vi "Process Incoming Messages by PDU F.vi"(0 "J1939 Cluster":T11, 1 "Scale Ref":T2, 2 "Data Ref":T1, 5 "CAN frame":T9 {"payload" format="%x"; "timestamp" format="%<%.7X\n%x>T"; "type" items=["CAN Data"=0, "CAN Remote"=1, "CAN Bus Error"=2, "CAN 2.0 Data"=8, "CAN FD Data"=16, "CAN FD+BRS Data"=24, "J1939 Data"=192, "Delay"=224, "Log Trigger"=225, "Start Trigger"=226]; "identifier" format="%x"}, 7 "ref in":T3, 9 "Addresses":u8[](array[numeric]), 11 "error in":errorcluster, 12 "Simulated Addresses LUT":variant) -> (15 "error out":errorcluster)   [LabVIEW 2015, in "J1939 Addon Engine.lvlib"]
uses:
  J1939 Addon Engine.lvlib
  Types/Setup Information Cluster.ctl
  <vilib>/xnet/xnet.llb/XNET Frame CAN.ctl
  <vilib>/xnet/xnet.llb/XNET Frame Type CAN.ctl
  Shared/J1939 Utilities/Types/CAN Outgoing Message Cluster.ctl
  Types/TP List References.ctl
  Types/BAM Buffer Connections List_Ref.ctl
  Types/TP Buffer Connection Cluster.ctl
  Types/Connection Mode Generation Connection Ref.ctl
  Types/Connection Mode Generation Connection Cluster.ctl
  Types/BAM Generation Connections List_Ref.ctl
  Types/BAM Generation Connection Cluster.ctl
  Types/Address Table Reference.ctl
  Types/RQST Lookup Table Reference.ctl
  Types/Conversion Lookup Table Reference.ctl
  Types/Data Lookup Table Reference.ctl
  Types/Datatable Lookup DVR.ctl
  Shared/J1939 Utilities/Types/PGN Fields Cluster.ctl
  Types/Simulated Settings.ctl
  Shared/Types/Compiled Simulated Settings.ctl
  Shared/Types/Monitor Settings.ctl
  <vilib>/NI Veristand/Custom Device API/Block Data Reference.ctl
  <vilib>/NI Veristand/Custom Device API/Data Reference.ctl
  Types/DTC FIFOs.ctl
  Types/TP Connections List State.ctl
  Types/Connection Mode Buffer Create New TP Connection State.ctl
  Types/Address Lookup Table Action.ctl
  Shared/Types/Address Lookup Table Data.ctl
  Shared/J1939 Utilities/SubVIs/Convert CAN Arb ID to J1939 ID.vi
  Shared/J1939 Utilities/SubVIs/Convert J1939 ID to CAN Arb ID.vi
  Shared/J1939 Utilities/SubVIs/Convert CAN Data (U32) to U8.vi
  Shared/J1939 Utilities/SubVIs/Acknowledgement.vi
  Buffer Connections List_Actions.vi
  TP Buffer Search for Connection (No PGN).vi
  TP Buffer Add New Data Packet to Connection.vi
  TP Buffer Convert Connection Info to CAN Frame.vi
  TP Buffer Create New TP Connection.vi
  Shared/J1939 Utilities/SubVIs/TP.CM EndofMsgACK.vi
  Shared/J1939 Utilities/SubVIs/TP.CM CTS.vi
  Shared/J1939 Utilities/SubVIs/TP.Conn Abort.vi
  Connection Mode Generation Connections List_Actions.vi
  Connection Mode Generation Search for Connection (Remote Message).vi
  TP Buffer Search for Connection.vi
  Connection Mode Generation CTS Received.vi
  Convert Data to DTC Frame.vi
  Conversion Lookup Table Get Conversion Parameter.vi
  Data Lookup Table Get Signals (Range).vi
  Shared/J1939 Utilities/SubVIs/Convert PGN + SA to J1939 ID.vi
  Address Lookup Table.vi
  BAM Buffer Connections List.vi
  Connection Mode Generation Connections List.vi
  <vilib>/xnet/xnet.llb/XNET Convert.vi
  <vilib>/xnet/xnet.llb/XNET Convert (Signal to Frame Raw).vi
  Data Lookup Table.vi
  Conversion Lookup Table.vi
  RQST Lookup Table.vi
  Shared/J1939 Utilities/J1939 Utilities.lvlib
  Shared/J1939 Addon Shared.lvlib
  <vilib>/NI VeriStand/Custom Device API/Custom Device API.lvlib
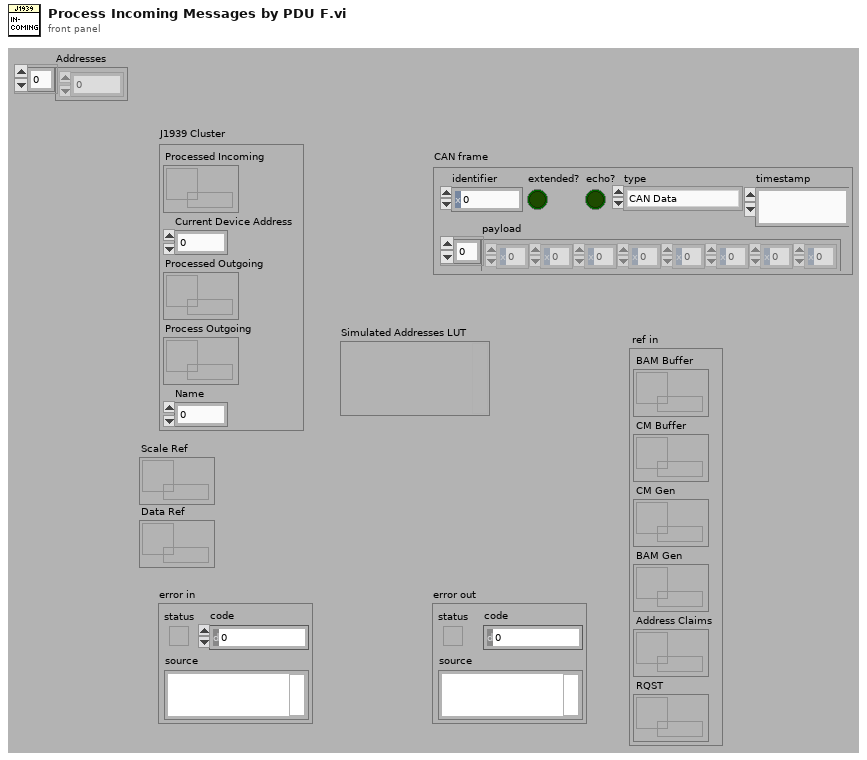
[diagram p1: front panel]
types:
  T1 = typedef "J1939 Addon Engine.lvlib/Data Lookup Table Reference.ctl" = refnum<data-value>
  T2 = typedef "J1939 Addon Engine.lvlib/Conversion Lookup Table Reference.ctl" = refnum<data-value>
  T3 = typedef "J1939 Addon Engine.lvlib/TP List References.ctl" = cluster{"BAM Buffer":T4, "CM Buffer":T4, "CM Gen":T5, "BAM Gen":T6, "Address Claims":T7, "RQST":T8}
  T4 = typedef "J1939 Addon Engine.lvlib/BAM Buffer Connections List_Ref.ctl" = refnum<data-value>
  T5 = typedef "J1939 Addon Engine.lvlib/Connection Mode Generation Connection Ref.ctl" = refnum<data-value>
  T6 = typedef "J1939 Addon Engine.lvlib/BAM Generation Connections List_Ref.ctl" = refnum<data-value>
  T7 = typedef "J1939 Addon Engine.lvlib/Address Table Reference.ctl" = refnum<data-value>
  T8 = typedef "J1939 Addon Engine.lvlib/RQST Lookup Table Reference.ctl" = refnum<data-value>
  T9 = typedef "XNET Frame CAN.ctl" = cluster{"timestamp":timestamp, "payload":u8[], "identifier":u32, "type":T10, "extended?":bool, "echo?":bool}
  T10 = typedef "XNET Frame Type CAN.ctl" = u8
  T11 = typedef "J1939 Addon Engine.lvlib/Setup Information Cluster.ctl" = cluster{"Processed Incoming":refnum<queue>, "Current Device Address":u8, "Processed Outgoing":refnum<queue>, "Process Outgoing":refnum<queue>, "Name":u64}
  T12 = typedef "J1939 Addon Shared.lvlib/J1939 Utilities.lvlib/Message Types.ctl" = enum8{"PDU 1", "RQST2", "XFER", "ACKM", "RQST", "TP.DT - RTS/CTS", "TP.DT - BAM", "TP.CM - RTS", "TP.CM - CTS", "TP.CM - EndofMsgACK", "TP.CM - BAM", "TP.CM - Abort", "TP.CM - Error", "ACL", "Proprietary A", "PDU 2", "Proprietary B", "Error"}
  T13 = typedef "J1939 Addon Engine.lvlib/Simulated Settings.ctl" = cluster{"Simulated Addresses":T14, "FIFOs":T18}
  T14 = typedef "J1939 Addon Shared.lvlib/Compiled Simulated Settings.ctl" = cluster{"J1939 XNET Settings":T15, "DM1 Data":T16[], "DM1 Data":dbl[], "DM1 Enable?":T16[], "DM1 Enable?":dbl[], "DM2 Data":T16[], "DM2 Data":dbl[], "DM2 Enable?":T16[], "DM2 Enable?":dbl[]}
  T15 = typedef "J1939 Addon Shared.lvlib/Monitor Settings.ctl" = cluster{"J1939 Network Address":u8, "Name":u64}
  T16 = typedef "Custom Device API.lvlib/Block Data Reference.ctl" = cluster{"Data Reference":T17, "Offset":u64, "Length":u64}
  T17 = typedef "Custom Device API.lvlib/Data Reference.ctl" = i32
  T18 = typedef "J1939 Addon Engine.lvlib/DTC FIFOs.ctl" = cluster{"DM1 Data":refnum<k33>, "DM1 Enable?":refnum<k33>, "DM2 Data":refnum<k33>, "DM2 Enable?":refnum<k33>, "DM1 Reset?":refnum<k33>, "DM2 Reset?":refnum<k33>}
  T19 = typedef "J1939 Addon Shared.lvlib/J1939 Utilities.lvlib/PGN Fields Cluster.ctl" = cluster{"Reserved Bit":u8, "Data page":u8, "PDU Format":u8, "PDU Specific":u8}
  T20 = typedef "J1939 Addon Shared.lvlib/J1939 Utilities.lvlib/CAN Outgoing Message Cluster.ctl" = cluster{"Identifier":u32, "Data":u8[]}
  T21 = typedef "J1939 Addon Engine.lvlib/TP Connections List State.ctl" = enum16{"Add", "Update", "Get", "Remove", "Initialize"}
  T22 = typedef "J1939 Addon Engine.lvlib/Connection Mode Buffer Create New TP Connection State.ctl" = enum8{"Find Connection", "Create Connection", "Create CTS Frame", "Abort New Connection"}
  T23 = typedef "J1939 Addon Shared.lvlib/Address Lookup Table Data.ctl" = cluster{"Name":u8[], "Address":u8}
  T24 = typedef "J1939 Addon Engine.lvlib/Address Lookup Table Action.ctl" = enum16{"Initialize", "Add", "Get", "Remove", "Get All"}
  T25 = typedef "J1939 Addon Engine.lvlib/RQST Lookup Table Cluster.ctl" = cluster{"Response Q":refnum<queue>, "Request PGN":u32}
  T26 = typedef "J1939 Addon Shared.lvlib/J1939 Utilities.lvlib/Convert CAN Data (U8) Cluster.ctl" = cluster{"Byte 1":u8, "Byte 2":u8, "Byte 3":u8, "Byte 4":u8, "Byte 5":u8, "Byte 6":u8, "Byte 7":u8, "Byte 8":u8}
  T27 = typedef "J1939 Addon Engine.lvlib/TP Buffer Connection Cluster.ctl" = cluster{"Source Address":u8, "Destination Address":u8, "PGN":u32, "Arb ID":u32, "CAN Conversion Index":u32, "Total Expected Bytes":u16, "Total Expected Packets":u8, "Number of Packets Read":u8, "Start Time":u32, "Packets (U8)":u8[], "Timestamp":timestamp}
  T28 = typedef "J1939 Addon Engine.lvlib/Connection Mode Generation Connection Cluster.ctl" = cluster{"Total Packets":u8, "Current Packet to Generate":u8, "Packets":T20[], "Previous Time Stamp":u32, "Total Bytes":u16, "Packet Identifier [PDU S + SA]":u16, "Number of Packets to Generate":u8, "PGN":u32}
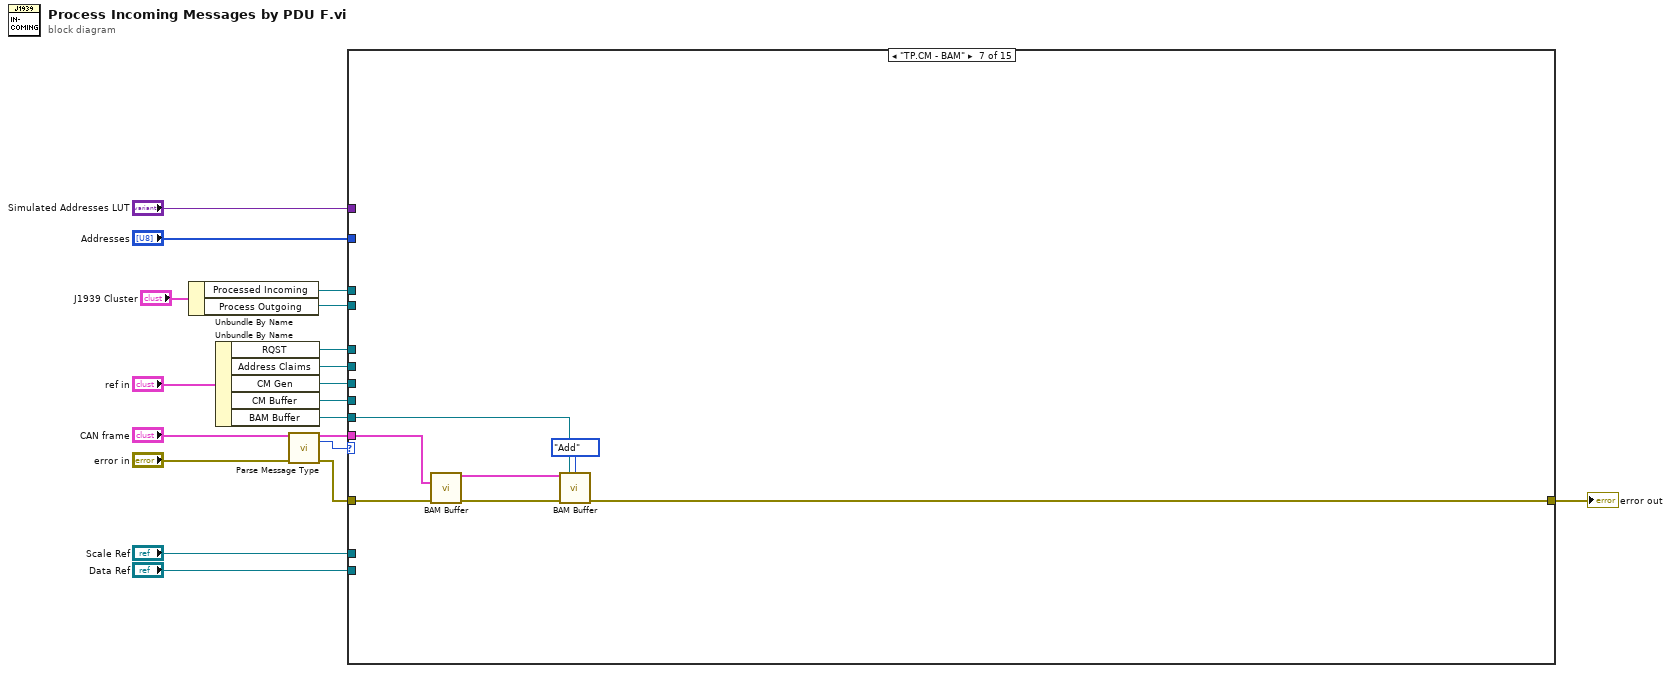
[diagram p0: block diagram]
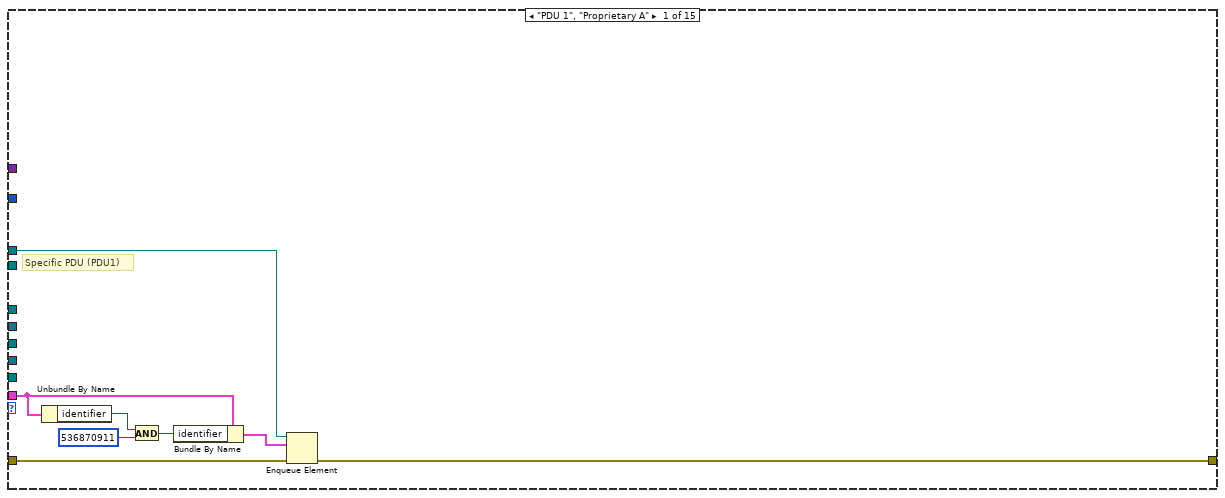
[diagram p2: hidden frame]
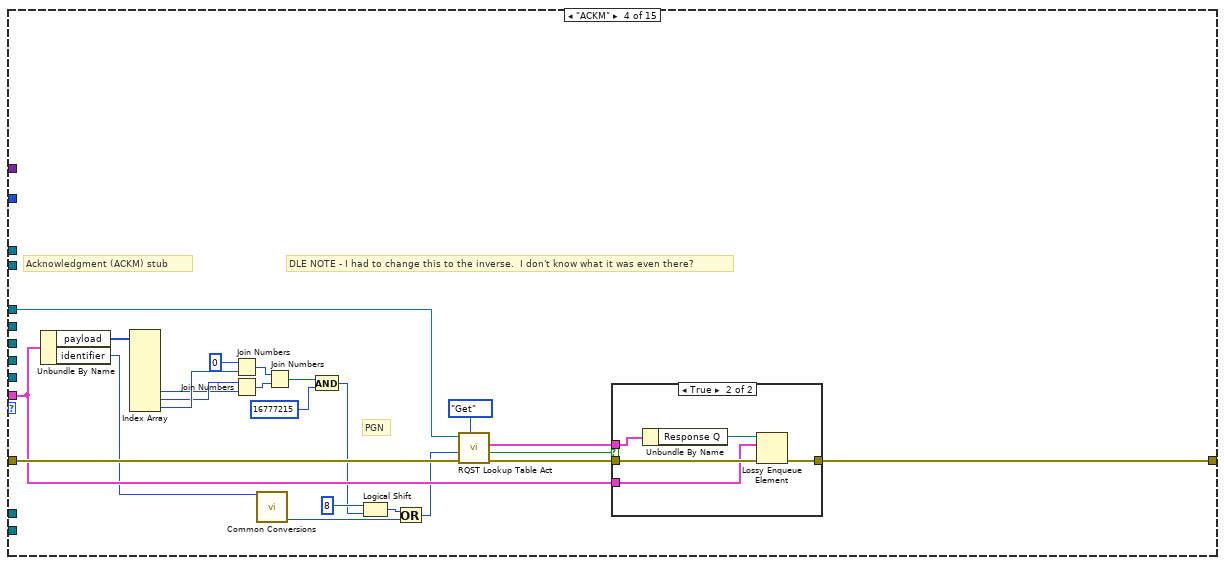
[diagram p5: hidden frame]
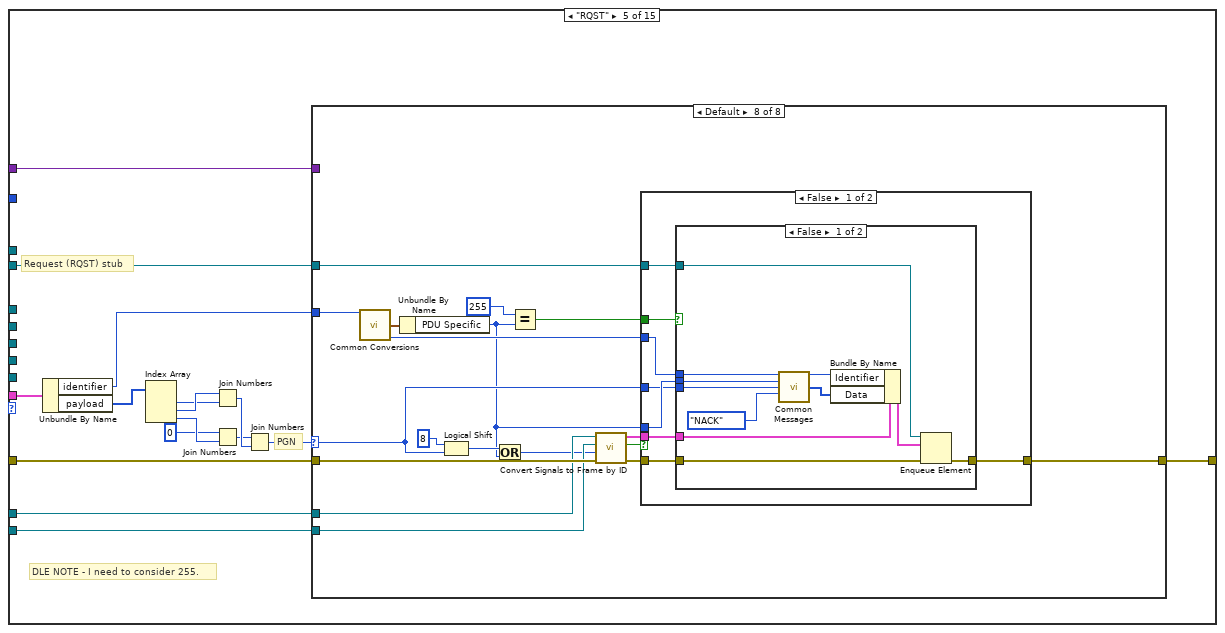
[diagram p7: hidden frame]
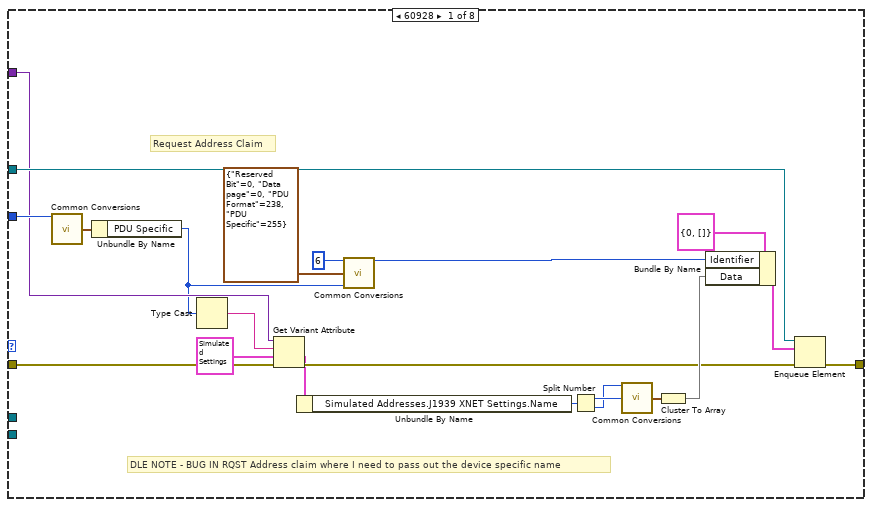
[diagram p8: hidden frame]
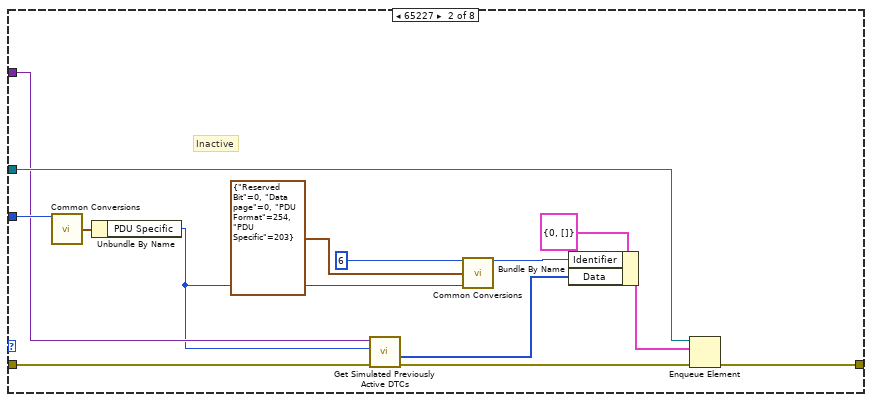
[diagram p9: hidden frame]
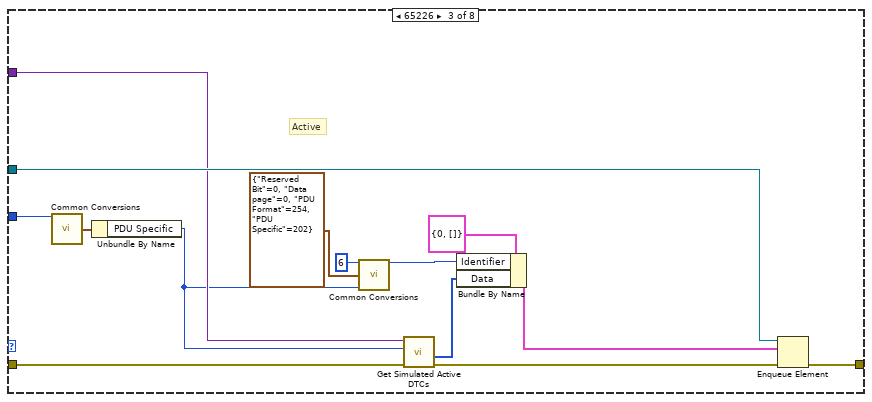
[diagram p10: hidden frame]
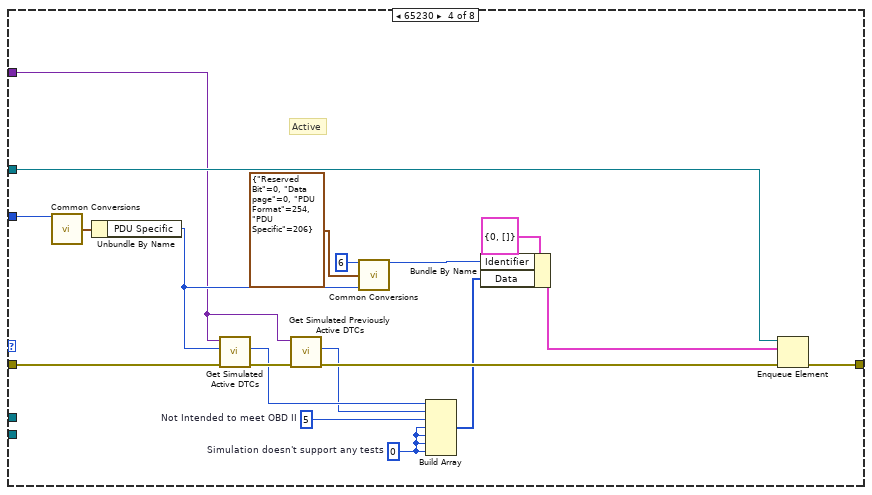
[diagram p11: hidden frame]
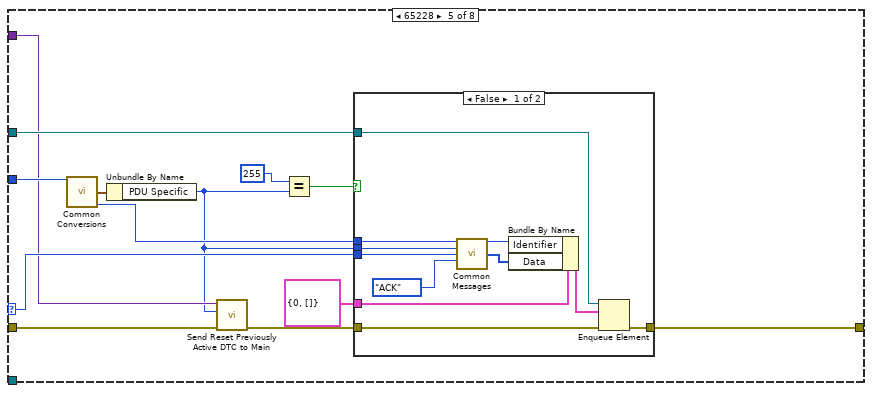
[diagram p12: hidden frame]
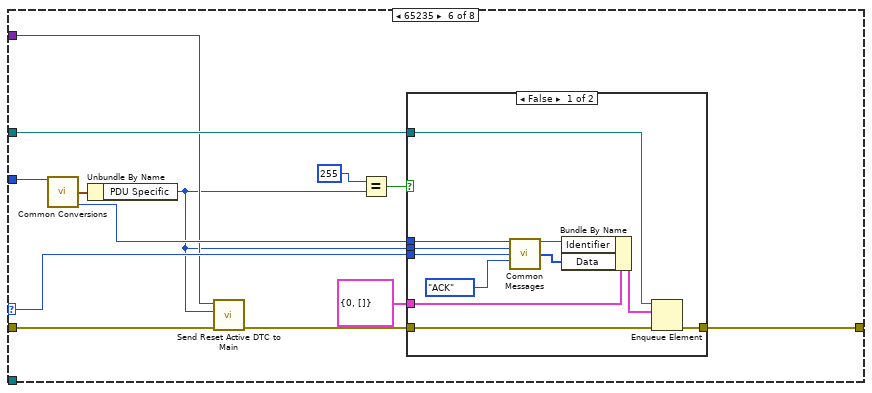
[diagram p14: hidden frame]
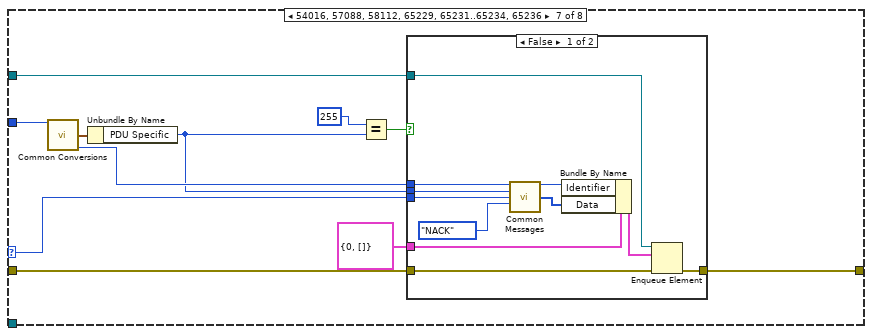
[diagram p16: hidden frame]
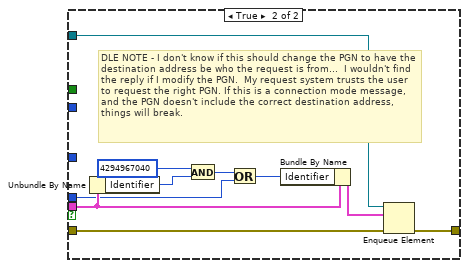
[diagram p19: hidden frame]
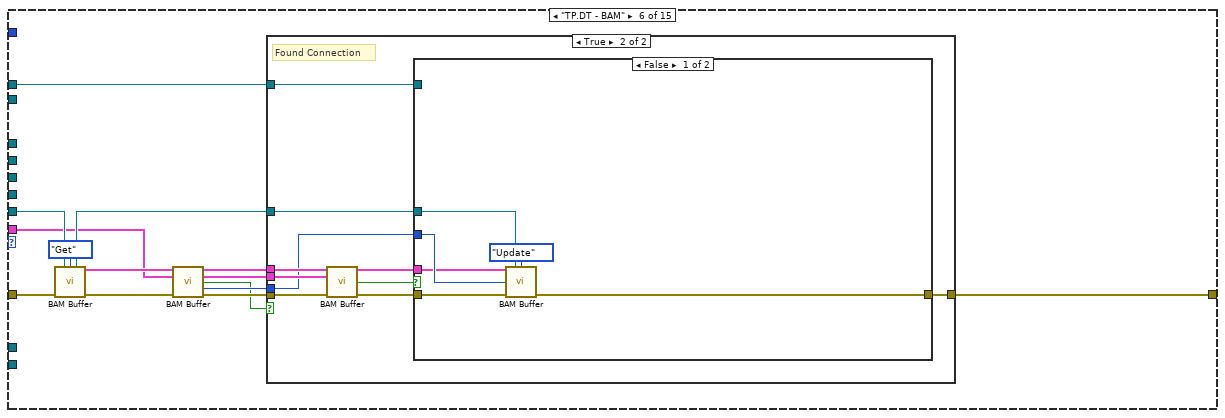
[diagram p20: hidden frame]
diagram:
  n1 = Unbundle By Name("J1939 Cluster") -> ("Processed Incoming"=w13:refnum<queue>, "Process Outgoing"=w12:refnum<queue>)
  n2 = Unbundle By Name("ref in") -> ("RQST"=w6:T8, "Address Claims"=w7:T7, "CM Gen"=w8:T5, "CM Buffer"=w9:T4, "BAM Buffer"=w10:T4)
  n3 = call "Parse Message Type.vi"("CAN frame"="CAN frame", "error in"="error in") -> ("CAN frame"=w16:T9, "State"=w15:T12, "error out"=w17:errorcluster)  [unwired: 1 in, 10 out]
  n4 = case shown="\"TP.CM - BAM\"" w15 {
    tunnel: w17 -> [w27 w28 w29 w39 w65 w270 w311 w327 w394 w496 w537 w553 w589 w601 w607]
    tunnel: [w26 w28 w29 w40 w66 w272 w308 w320 w393 w495 w536 w554 w582 w602 w607] -> w19
    tunnel: w16 -> [w22 _ _ w38 w74 w264 w305 w314 w390 w484 w527 w544 w580 w599 _]
    tunnel: w13 -> [w25 _ _ _ _ w267 _ w318 _ _ _ _ w579 w600 _]
    tunnel: w12 -> [_ _ _ _ w64 _ _ w317 w392 _ _ _ _ _ _]
    tunnel: w10 -> [_ _ _ _ _ w266 w306 _ _ _ _ _ _ _ _]
    tunnel: w9 -> [_ _ _ _ _ _ _ w316 w391 w483 _ w547 _ _ _]
    tunnel: w8 -> [_ _ _ _ _ _ _ _ _ w486 w529 w545 _ _ _]
    tunnel: w7 -> [_ _ _ _ _ _ _ _ _ _ _ _ w587 _ _]
    tunnel: w6 -> [_ _ _ w30 _ _ _ _ _ _ _ _ _ _ _]
    tunnel: "Scale Ref" -> [_ _ _ _ w62 _ _ _ _ _ _ _ _ _ _]
    tunnel: "Data Ref" -> [_ _ _ _ w61 _ _ _ _ _ _ _ _ _ _]
    tunnel: "Addresses" -> [_ _ _ _ _ _ _ w312 w389 _ _ _ _ _ _]
    tunnel: "Simulated Addresses LUT" -> [_ _ _ _ w59 _ _ _ _ _ _ _ _ _ _]
    frame "PDU 1", "Proprietary A" {
      # "Specific PDU (PDU1)"
      n5 = Unbundle By Name(w22) -> ("identifier"=w24:u32)
      n6 = And(x=w24, y=u32 536870911) -> (x .and. y?=w20:u32)
      n7 = Bundle By Name(cluster=w22, "identifier"=w20) -> (w21:T9)
      n8 = Enqueue Element(queue=w25, element=w21, error in (no error)=w27) -> (error out=w26:errorcluster)  [unwired: 3 out]
    }
    frame "RQST2" {
      # "Request2 (RQST2) Stub"
    }
    frame "XFER" {
      # "Transfer (XFER) Stub"
    }
    frame "ACKM" {
      # "DLE NOTE - I had to change this to the inverse.  I don't know what it was even there?"
      # "PGN"
      # "Acknowledgment (ACKM) stub"
      n9 = Unbundle By Name(w38) -> ("payload"=w52:u8[], "identifier"=w35:u32)
      n10 = Index Array(array=w52) -> (element #6=w49:u8, element #7=w50:u8, element #8=w51:u8)  [unwired: 8 in, 5 out]
      n11 = Join Numbers(hi=u8 0, lo=w51) -> ((hi.lo)=w48:u16)
      n12 = Join Numbers(hi=w50, lo=w49) -> ((hi.lo)=w47:u16)
      n13 = call-poly "Common Conversions.vi"("Arb ID"=w35) -> ("Source Address"=w34:u8)  [unwired: 11 in, 3 out]
      n14 = Join Numbers(hi=w48, lo=w47) -> ((hi.lo)=w46:u32)
      n15 = And(x=w46, y=u32 16777215 ("x")) -> (x .and. y?=w33:u32)
      n16 = Logical Shift(y=i8 8, x=w33) -> (x << y=w37:u32)
      n17 = Or(x=w37, y=w34) -> (x .or. y?=w32:u32)
      n18 = call "RQST Lookup Table Act.vi"("Action"=enum16{"Initialize", "Add", "Get", "Remove"}."Get", "error in (no error)"=w39, "ID"=w32, "Rqst LUT"=w30) -> ("error out"=w31:errorcluster, "Found?"=w42:bool, "Data"=w41:T25)  [unwired: 4 in, 1 out]
      n19 = case shown="True" w42 {
        tunnel: w41 -> [_ w57]
        tunnel: w31 -> [w53 w58]
        tunnel: w38 -> [_ w55]
        tunnel: [w53 w54] -> w40
        frame False {
        }
        frame True {
          n20 = Unbundle By Name(w57) -> ("Response Q"=w56:refnum<queue>)
          n21 = Lossy Enqueue Element(queue=w56, element=w55, error in (no error)=w58) -> (error out=w54:errorcluster)  [unwired: 3 out]
        }
      }
    }
    frame "RQST" {
      # "DLE NOTE - I need to consider 255."
      # "PGN"
      # "Request (RQST) stub"
      n22 = Unbundle By Name(w74) -> ("identifier"=w63:u32, "payload"=w73:u8[])
      n23 = Index Array(array=w73) -> (element #1=w60:u8, element #2=w72:u8, element #3=w71:u8)  [unwired: 3 in]
      n24 = Join Numbers(hi=w72, lo=w60) -> ((hi.lo)=w69:u16)
      n25 = Join Numbers(hi=u8 0, lo=w71) -> ((hi.lo)=w68:u16)
      n26 = Join Numbers(hi=w68, lo=w69) -> ((hi.lo)=w67:u32)
      n27 = case shown="Default" w67 {
        selector: w67 -> [_ _ _ _ w149 w174 w197 w223]
        tunnel: [w91 w102 w117 w136 w150 w172 w195 w224] -> w66
        tunnel: w65 -> [w78 w98 w111 w132 w146 w171 w193 w233]
        tunnel: w64 -> [w89 w101 w116 w135 w151 w175 w198 w225]
        tunnel: w63 -> [w83 w108 w122 w141 w154 w173 w196 w226]
        tunnel: w62 -> [_ _ _ _ _ _ _ w232]
        tunnel: w61 -> [_ _ _ _ _ _ _ w231]
        tunnel: w59 -> [w80 w100 w113 w129 w144 w169 _ _]
        frame 60928 {
          # "DLE NOTE - BUG IN RQST Address claim where I need to pass out the device specific name"
          # "Request Address Claim"
          n28 = call-poly "Common Conversions.vi"("Arb ID"=w83) -> ("PGN Fields"=w84:T19)  [unwired: 11 in, 3 out]
          n29 = Unbundle By Name(w84) -> ("PDU Specific"=w79:u8)
          n30 = Type Cast(x=w79) -> (*(type *) &x=w81:string)  [unwired: 1 in]
          n31 = Get Variant Attribute(Variant=w80, name=w81, default value (empty Variant)=T13 {"Simulated Addresses"={"J1939 XNET Settings"={"J1939 Network Address"=0, "Name"=0}, "DM1 Data"=[], "DM1 Data"=[], "DM1 Enable?"=[], "DM1 Enable?"=[], "DM2 Data"=[], "DM2 Data"=[], "DM2 Enable?"=[], "DM2 Enable?"=[]}, "FIFOs"={"DM1 Data"=refnum, "DM1 Enable?"=refnum, "DM2 Data"=refnum, "DM2 Enable?"=refnum, "DM1 Reset?"=refnum, "DM2 Reset?"=refnum}} ("Cluster"), error in=w78) -> (value=w76:T13, error out=w77:errorcluster)  [unwired: 2 out]
          n32 = Unbundle By Name(w76) -> ("Simulated Addresses.J1939 XNET Settings.Name"=w75:u64)
          n33 = call-poly "Common Conversions.vi"("Priority"=u8 6, "PGN Fields"=T19 {"Reserved Bit"=0, "Data page"=0, "PDU Format"=238, "PDU Specific"=255}, "Source Address"=w79) -> ("ID"=w93:u32)  [unwired: 2 in, 10 out]
          n34 = Split Number(x=w75) -> (hi(x)=w87:u32, lo(x)=w86:u32)
          n35 = call-poly "Common Conversions.vi"("Data 0-3"=w86, "Data 4-7"=w87) -> ("Byte Cluster"=w88:T26)  [unwired: 13 in]
          n36 = Cluster To Array(cluster=w88) -> (array=w85:u8[])
          n37 = Bundle By Name(cluster=T20 {"Identifier"=0, "Data"=[]} ("Data to Send"), "Identifier"=w93, "Data"=w85) -> (w90:T20)
          n38 = Enqueue Element(queue=w89, element=w90, error in (no error)=w77) -> (error out=w91:errorcluster)  [unwired: 1 in, 2 out]
        }
        frame 65227 {
          # "Inactive"
          n39 = call-poly "Common Conversions.vi"("Arb ID"=w108) -> ("PGN Fields"=w109:T19)  [unwired: 11 in, 3 out]
          n40 = Unbundle By Name(w109) -> ("PDU Specific"=w99:u8)
          n41 = call "Get Simulated Previously Active DTCs.vi"("error in (no error)"=w98, "Address"=w99, "Simulated Addresses LUT"=w100) -> ("error out"=w97:errorcluster, "DTC Frame"=w96:u8[])  [unwired: 5 in, 2 out]
          n42 = call-poly "Common Conversions.vi"("Priority"=u8 6, "PGN Fields"=T19 {"Reserved Bit"=0, "Data page"=0, "PDU Format"=254, "PDU Specific"=203}, "Source Address"=w99) -> ("ID"=w105:u32)  [unwired: 2 in, 10 out]
          n43 = Bundle By Name(cluster=T20 {"Identifier"=0, "Data"=[]} ("Data to Send"), "Identifier"=w105, "Data"=w96) -> (w107:T20)
          n44 = Enqueue Element(queue=w101, element=w107, error in (no error)=w97) -> (error out=w102:errorcluster)  [unwired: 1 in, 2 out]
        }
        frame 65226 {
          # "Active"
          n45 = call-poly "Common Conversions.vi"("Arb ID"=w122) -> ("PGN Fields"=w123:T19)  [unwired: 11 in, 3 out]
          n46 = Unbundle By Name(w123) -> ("PDU Specific"=w112:u8)
          n47 = call-poly "Common Conversions.vi"("Priority"=u8 6, "PGN Fields"=T19 {"Reserved Bit"=0, "Data page"=0, "PDU Format"=254, "PDU Specific"=202}, "Source Address"=w112) -> ("ID"=w119:u32)  [unwired: 2 in, 10 out]
          n48 = call "Get Simulated Active DTCs.vi"("error in (no error)"=w111, "Address"=w112, "Simulated Addresses LUT"=w113) -> ("error out"=w114:errorcluster, "DTC Frame"=w110:u8[])  [unwired: 5 in, 2 out]
          n49 = Bundle By Name(cluster=T20 {"Identifier"=0, "Data"=[]} ("Data to Send"), "Identifier"=w119, "Data"=w110) -> (w121:T20)
          n50 = Enqueue Element(queue=w116, element=w121, error in (no error)=w114) -> (error out=w117:errorcluster)  [unwired: 1 in, 2 out]
        }
        frame 65230 {
          w125 = u8 0  # Simulation doesn't support any tests
          w126 = u8 5  # Not Intended to meet OBD II
          # "Active"
          n51 = call-poly "Common Conversions.vi"("Arb ID"=w141) -> ("PGN Fields"=w142:T19)  [unwired: 11 in, 3 out]
          n52 = Unbundle By Name(w142) -> ("PDU Specific"=w133:u8)
          n53 = call "Get Simulated Active DTCs.vi"("error in (no error)"=w132, "Address"=w133, "Simulated Addresses LUT"=w129) -> ("error out"=w131:errorcluster, "# of Enabled"=w128:u8)  [unwired: 5 in, 2 out]
          n54 = call "Get Simulated Previously Active DTCs.vi"("error in (no error)"=w131, "Simulated Addresses LUT"=w129) -> ("error out"=w130:errorcluster, "# of Enabled"=w127:u8)  [unwired: 6 in, 2 out]
          n55 = call-poly "Common Conversions.vi"("Priority"=u8 6, "PGN Fields"=T19 {"Reserved Bit"=0, "Data page"=0, "PDU Format"=254, "PDU Specific"=206}, "Source Address"=w133) -> ("ID"=w138:u32)  [unwired: 2 in, 10 out]
          n56 = Build Array(w128, w127, w126, w125, w125, w125, w125) -> (w124:u8[])
          n57 = Bundle By Name(cluster=T20 {"Identifier"=0, "Data"=[]} ("Data to Send"), "Identifier"=w138, "Data"=w124) -> (w140:T20)
          n58 = Enqueue Element(queue=w135, element=w140, error in (no error)=w130) -> (error out=w136:errorcluster)  [unwired: 1 in, 2 out]
        }
        frame 65228 {
          n59 = call-poly "Common Conversions.vi"("Arb ID"=w154) -> ("PGN Fields"=w155:T19, "Source Address"=w148:u8)  [unwired: 11 in, 2 out]
          n60 = Unbundle By Name(w155) -> ("PDU Specific"=w143:u8)
          n61 = call "Send Reset Previously Active DTC to Main.vi"("error in (no error)"=w146, "Address"=w143, "Simulated Addresses LUT"=w144) -> ("error out"=w145:errorcluster)  [unwired: 7 in, 1 out]
          n62 = Equal?(x=u8 255 ("y"), y=w143) -> (x = y?=w152:bool)
          n63 = case shown="False" w152 {
            tunnel: w145 -> [w166 w167]
            tunnel: [w165 w167] -> w150
            tunnel: w151 -> [w164 _]
            tunnel: w148 -> [w163 _]
            tunnel: w143 -> [w162 _]
            tunnel: w149 -> [w161 _]
            tunnel: T20 {"Identifier"=0, "Data"=[]} ("Frame") -> [w159 _]
            frame False {
              n64 = call-poly "Common Messages.vi"("Destination Address"=w163, "Source Address"=w162, "PGN"=w161, "Control Byte"=enum8{"ACK", "NACK", "Access Denied"}."ACK") -> ("Arb ID"=w158:u32, "Data"=w157:u8[])  [unwired: 10 in]
              n65 = Bundle By Name(cluster=w159, "Identifier"=w158, "Data"=w157) -> (w156:T20)
              n66 = Enqueue Element(queue=w164, element=w156, error in (no error)=w166) -> (error out=w165:errorcluster)  [unwired: 3 out]
            }
            frame True {
            }
          }
        }
        frame 65235 {
          n67 = call-poly "Common Conversions.vi"("Arb ID"=w173) -> ("PGN Fields"=w180:T19, "Source Address"=w177:u8)  [unwired: 11 in, 2 out]
          n68 = Unbundle By Name(w180) -> ("PDU Specific"=w168:u8)
          n69 = call "Send Reset Active DTC to Main.vi"("error in (no error)"=w171, "Address"=w168, "Simulated Addresses LUT"=w169) -> ("error out"=w170:errorcluster)  [unwired: 7 in, 1 out]
          n70 = Equal?(x=u8 255 ("y"), y=w168) -> (x = y?=w178:bool)
          n71 = case shown="False" w178 {
            tunnel: w170 -> [w191 w192]
            tunnel: [w190 w192] -> w172
            tunnel: w175 -> [w189 _]
            tunnel: w177 -> [w188 _]
            tunnel: w168 -> [w187 _]
            tunnel: w174 -> [w186 _]
            tunnel: T20 {"Identifier"=0, "Data"=[]} ("Frame") -> [w184 _]
            frame False {
              n72 = call-poly "Common Messages.vi"("Destination Address"=w188, "Source Address"=w187, "PGN"=w186, "Control Byte"=enum8{"ACK", "NACK", "Access Denied"}."ACK") -> ("Arb ID"=w183:u32, "Data"=w182:u8[])  [unwired: 10 in]
              n73 = Bundle By Name(cluster=w184, "Identifier"=w183, "Data"=w182) -> (w181:T20)
              n74 = Enqueue Element(queue=w189, element=w181, error in (no error)=w191) -> (error out=w190:errorcluster)  [unwired: 3 out]
            }
            frame True {
            }
          }
        }
        frame 54016, 57088, 58112, 65229, 65231..65234, 65236 {
          n75 = call-poly "Common Conversions.vi"("Arb ID"=w196) -> ("PGN Fields"=w203:T19, "Source Address"=w200:u8)  [unwired: 11 in, 2 out]
          n76 = Unbundle By Name(w203) -> ("PDU Specific"=w194:u8)
          n77 = Equal?(x=u8 255 ("y"), y=w194) -> (x = y?=w201:bool)
          n78 = case shown="False" w201 {
            tunnel: w193 -> [w214 w215]
            tunnel: [w213 w215] -> w195
            tunnel: w198 -> [w212 _]
            tunnel: w200 -> [w211 _]
            tunnel: w194 -> [w210 _]
            tunnel: w197 -> [w209 _]
            tunnel: T20 {"Identifier"=0, "Data"=[]} ("Frame") -> [w207 _]
            frame False {
              n79 = call-poly "Common Messages.vi"("Destination Address"=w211, "Source Address"=w210, "PGN"=w209, "Control Byte"=enum8{"ACK", "NACK", "Access Denied"}."NACK") -> ("Arb ID"=w206:u32, "Data"=w205:u8[])  [unwired: 10 in]
              n80 = Bundle By Name(cluster=w207, "Identifier"=w206, "Data"=w205) -> (w204:T20)
              n81 = Enqueue Element(queue=w212, element=w204, error in (no error)=w214) -> (error out=w213:errorcluster)  [unwired: 3 out]
            }
            frame True {
            }
          }
        }
        frame Default {
          n82 = call-poly "Common Conversions.vi"("Arb ID"=w226) -> ("PGN Fields"=w222:T19, "Source Address"=w219:u8)  [unwired: 11 in, 2 out]
          n83 = Unbundle By Name(w222) -> ("PDU Specific"=w216:u8)
          n84 = Logical Shift(y=i8 8, x=w223) -> (x << y=w218:u32)
          n85 = Or(x=w218, y=w216) -> (x .or. y?=w217:u32)
          n86 = Equal?(x=u8 255 ("y"), y=w216) -> (x = y?=w220:bool)
          n87 = call "Convert Signals to Frame by ID.vi"("error in (no error)"=w233, "ID"=w217, "Data Ref"=w231, "Scale Ref"=w232) -> ("error out"=w227:errorcluster, "Found?"=w228:bool, "Frame"=w229:T20)  [unwired: 5 in]
          n88 = case shown="False" w228 {
            tunnel: w229 -> [w235 w263]
            tunnel: w216 -> [w237 w261]
            tunnel: [w240 w256] -> w224
            tunnel: w227 -> [w241 w257]
            tunnel: w219 -> [w238 _]
            tunnel: w225 -> [w239 w258]
            tunnel: w223 -> [w236 _]
            tunnel: w220 -> [w234 _]
            frame False {
              n89 = case shown="False" w234 {
                tunnel: w241 -> [w252 w253]
                tunnel: [w251 w253] -> w240
                tunnel: w239 -> [w250 _]
                tunnel: w238 -> [w249 _]
                tunnel: w237 -> [w248 _]
                tunnel: w236 -> [w247 _]
                tunnel: w235 -> [w245 _]
                frame False {
                  n90 = call-poly "Common Messages.vi"("Destination Address"=w249, "Source Address"=w248, "PGN"=w247, "Control Byte"=enum8{"ACK", "NACK", "Access Denied"}."NACK") -> ("Arb ID"=w244:u32, "Data"=w243:u8[])  [unwired: 10 in]
                  n91 = Bundle By Name(cluster=w245, "Identifier"=w244, "Data"=w243) -> (w242:T20)
                  n92 = Enqueue Element(queue=w250, element=w242, error in (no error)=w252) -> (error out=w251:errorcluster)  [unwired: 3 out]
                }
                frame True {
                }
              }
            }
            frame True {
              # "DLE NOTE - I don't know if this should change the PGN to have the destination address be who the request is from...  I wouldn't find the reply if I modify the PGN.  My request system trusts the user to request the right PGN. If this is a connection mode message, and the PGN doesn't include the correct destination address, things will break."
              n93 = Unbundle By Name(w263) -> ("Identifier"=w262:u32)
              n94 = And(x=u32 4294967040 ("y"), y=w262) -> (x .and. y?=w254:u32)
              n95 = Or(x=w254, y=w261) -> (x .or. y?=w260:u32)
              n96 = Bundle By Name(cluster=w263, "Identifier"=w260) -> (w259:T20)
              n97 = Enqueue Element(queue=w258, element=w259, error in (no error)=w257) -> (error out=w256:errorcluster)  [unwired: 3 out]
            }
          }
        }
      }
    }
    frame "TP.DT - BAM" {
      n98 = call-poly "BAM Buffer.vi"("Connections Ref"=w266, "State"=TP_Connections_List_State."Get", "error in (no error)"=w270) -> ("Connections Ref out"=w265:T4, "Connections"=w276:T27[], "error out"=w269:errorcluster)  [unwired: 2 in, 8 out]
      n99 = call-poly "BAM Buffer.vi"("Connecctions"=w276, "CAN frame"=w264, "error in (no error)"=w269) -> ("Connection Cluster Out"=w275:T27, "CAN frame Out"=w274:T9, "Found?"=w268:bool, "Index"=w271:i32, "error out"=w273:errorcluster)  [unwired: 8 out]
      n100 = case shown="True" w268 {
        tunnel: w275 -> [_ w288]
        tunnel: w274 -> [_ w286]
        tunnel: w273 -> [w278 w285]
        tunnel: [w278 w283] -> w272
        tunnel: w271 -> [_ w282]
        tunnel: w267 -> [_ w280]
        tunnel: w265 -> [_ w279]
        frame False {
        }
        frame True {
          # "Found Connection"
          n101 = call-poly "BAM Buffer.vi"("Connection Cluster"=w288, "CAN frame"=w286, "error in (no error)"=w285) -> ("Connection Cluster Out"=w281:T27, "Message Complete?"=w287:bool, "error out"=w284:errorcluster)  [unwired: 10 out]
          n102 = case shown="False" w287 {
            tunnel: w284 -> [w292 w302]
            tunnel: [w291 w300] -> w283
            tunnel: w282 -> [w293 w303]
            tunnel: w281 -> [w289 w301]
            tunnel: w280 -> [_ w297]
            tunnel: w279 -> [w290 w295]
            frame False {
              n103 = call-poly "BAM Buffer.vi"("Connection Cluster"=w289, "Connections Ref"=w290, "State"=TP_Connections_List_State."Update", "index"=w293, "error in (no error)"=w292) -> ("error out"=w291:errorcluster)  [unwired: 7 in, 3 out]
            }
            frame True {
              n104 = call-poly "BAM Buffer.vi"("Connection Cluster"=w301, "error in (no error)"=w302) -> ("CAN frame"=w296:T9, "error out"=w299:errorcluster)  [unwired: 12 out]
              n105 = Enqueue Element(queue=w297, element=w296, error in (no error)=w299) -> (error out=w298:errorcluster)  [unwired: 3 out]
              n106 = call-poly "BAM Buffer.vi"("Connections Ref"=w295, "State"=TP_Connections_List_State."Remove", "index"=w303, "error in (no error)"=w298) -> ("error out"=w300:errorcluster)  [unwired: 1 in, 10 out]
            }
          }
        }
      }
    }
    frame "TP.CM - BAM" {
      n107 = call-poly "BAM Buffer.vi"("CAN frame"=w305, "error in (no error)"=w311) -> ("Connection Cluster Out"=w307:T27, "error out"=w309:errorcluster)  [unwired: 1 in, 11 out]
      n108 = call-poly "BAM Buffer.vi"("Connection Cluster"=w307, "Connections Ref"=w306, "State"=TP_Connections_List_State."Add", "error in (no error)"=w309) -> ("error out"=w308:errorcluster)  [unwired: 1 in, 10 out]
    }
    frame "TP.DT - RTS/CTS" {
      n109 = call-poly "Connnection Mode Buffer.vi"("Connections Ref"=w316, "State"=TP_Connections_List_State."Get", "error in (no error)"=w327) -> ("Connections Ref out"=w315:T4, "Connections"=w325:T27[], "error out"=w324:errorcluster)  [unwired: 2 in, 8 out]
      n110 = call-poly "Connnection Mode Buffer.vi"("Connecctions"=w325, "CAN frame"=w314, "error in (no error)"=w324) -> ("Connection Cluster Out"=w322:T27, "CAN frame Out"=w319:T9, "Found?"=w313:bool, "Index"=w321:i32, "error out"=w323:errorcluster)  [unwired: 8 out]
      n111 = case shown="True" w313 {
        tunnel: w323 -> [w328 w341]
        tunnel: w322 -> [_ w340]
        tunnel: w319 -> [_ w339]
        tunnel: w321 -> [_ w336]
        tunnel: [w328 w335] -> w320
        tunnel: w318 -> [_ w334]
        tunnel: w317 -> [_ w331]
        tunnel: w315 -> [_ w330]
        tunnel: w312 -> [_ w329]
        frame False {
        }
        frame True {
          # "Found Connection"
          n112 = call-poly "Connnection Mode Buffer.vi"("Connection Cluster"=w340, "CAN frame"=w339, "error in (no error)"=w341) -> ("Connection Cluster Out"=w337:T27, "Frame Mismatch?"=w332:bool, "Message Complete?"=w333:bool, "error out"=w338:errorcluster)  [unwired: 9 out]
          n113 = case shown="True" w333 {
            tunnel: w338 -> [w347 w367]
            tunnel: [w346 w374] -> w335
            tunnel: w336 -> [w345 w373]
            tunnel: w337 -> [w344 w366]
            tunnel: w334 -> [_ w369]
            tunnel: w332 -> [w343 _]
            tunnel: w331 -> [_ w360]
            tunnel: w330 -> [w342 w359]
            tunnel: w329 -> [_ w357]
            frame False {
              n114 = case shown="False" w343 {
                tunnel: w347 -> [w352 w354]
                tunnel: [w351 w354] -> w346
                tunnel: w345 -> [w350 _]
                tunnel: w344 -> [w349 _]
                tunnel: w342 -> [w348 _]
                frame False {
                  n115 = call-poly "Connnection Mode Buffer.vi"("Connection Cluster"=w349, "Connections Ref"=w348, "State"=TP_Connections_List_State."Update", "index"=w350, "error in (no error)"=w352) -> ("error out"=w351:errorcluster)  [unwired: 10 out]
                }
                frame True {
                }
              }
            }
            frame True {
              n116 = Unbundle By Name(w366) -> ("Source Address"=w365:u8, "Destination Address"=w356:u8, "PGN"=w364:u32, "Total Expected Bytes"=w362:u16, "Number of Packets Read"=w363:u8)
              n117 = Search 1D Array(1D array=w357, element=w356) -> (index of element=w355:i32)  [unwired: 1 in]
              n118 = Greater Or Equal To 0?(x=w355) -> (x >= 0?=w358:bool)
              n119 = case shown="True" w358 {
                tunnel: w367 -> [w375 w388]
                tunnel: w365 -> [_ w387]
                tunnel: w364 -> [_ w386]
                tunnel: w363 -> [_ w385]
                tunnel: w362 -> [_ w384]
                tunnel: [w375 w380] -> w361
                tunnel: w360 -> [_ w379]
                tunnel: w356 -> [_ w376]
                frame False {
                }
                frame True {
                  # "Only send if message was intended for our address."
                  n120 = call-poly "Connnection Mode Buffer.vi"("PGN"=w386, "Source Address"=w376, "Destination Address"=w387, "Total Message Size(bytes)"=w384, "Total Number of Packets"=w385, "error in (no error)"=w388) -> ("Arb ID"=w383:u32, "Data"=w382:u8[], "error out"=w381:errorcluster)  [unwired: 7 out]
                  n121 = Bundle(cluster=T20 {"Identifier"=0, "Data"=[]} ("Data to Send"), "Identifier"=w383, "Data"=w382) -> (w377:T20)
                  n122 = Enqueue Element(queue=w379, element=w377, error in (no error)=w381) -> (error out=w380:errorcluster)  [unwired: 3 out]
                }
              }
              n123 = call-poly "Connnection Mode Buffer.vi"("Connection Cluster"=w366, "error in (no error)"=w361) -> ("CAN frame"=w368:T9, "error out"=w371:errorcluster)  [unwired: 12 out]
              n124 = Enqueue Element(queue=w369, element=w368, error in (no error)=w371) -> (error out=w370:errorcluster)  [unwired: 3 out]
              n125 = call-poly "Connnection Mode Buffer.vi"("Connections Ref"=w359, "State"=TP_Connections_List_State."Remove", "index"=w373, "error in (no error)"=w370) -> ("error out"=w374:errorcluster)  [unwired: 1 in, 10 out]
            }
          }
        }
      }
    }
    frame "TP.CM - RTS" {
      n126 = while {
        shift-right: [w400] -> _
        shift-left: Connection_Mode_Buffer_Create_New_TP_Connection_State."Find Connection" ("Action") -> [w407]
        tunnel: w390 -> [w408]
        shift-right: [w405] -> _
        shift-left: _ -> [w399]
        shift-right: [w404] -> _
        shift-left: _ -> [w401]
        shift-right: [w403] -> w393
        shift-left: w394 -> [w406]
        tunnel: w392 -> [w398]
        tunnel: w391 -> [w397]
        tunnel: w389 -> [w396]
        stop <- w402 stop-if-true
        n127 = case shown="\"Create CTS Frame\"" w407 {
          selector: w407 -> [_ _ w446 w465]
          tunnel: w408 -> [w419 w432 _ w464]
          tunnel: w406 -> [w418 w434 w449 w463]
          tunnel: [w417 w428 w448 w470] -> w405
          tunnel: [w416 w437 w447 w468] -> w404
          tunnel: [w415 w435 w443 w467] -> w403
          tunnel: [FALSE w427 TRUE TRUE] -> w402
          tunnel: w401 -> [_ w437 w447 w468]
          tunnel: [w411 Connection_Mode_Buffer_Create_New_TP_Connection_State."Create CTS Frame" ("Action") w446 w465] -> w400
          tunnel: w399 -> [_ _ w448 w470]
          tunnel: w398 -> [_ _ w442 w466]
          tunnel: w397 -> [w409 w429 _ _]
          tunnel: w396 -> [_ w425 _ w457]
          frame "Find Connection" {
            n128 = call-poly "Connnection Mode Buffer.vi"("Connections Ref"=w409, "State"=TP_Connections_List_State."Get", "error in (no error)"=w418) -> ("Connections"=w421:T27[], "error out"=w422:errorcluster)  [unwired: 2 in, 9 out]
            n129 = call-poly "Connnection Mode Buffer.vi"("Connecctions"=w421, "CAN frame"=w419, "error in (no error)"=w422) -> ("Connection Cluster Out"=w417:T27, "Found?"=w412:bool, "Index"=w416:i32, "error out"=w415:errorcluster)  [unwired: 9 out]
            n130 = Select(t=Connection_Mode_Buffer_Create_New_TP_Connection_State."Abort New Connection", s=w412, f=Connection_Mode_Buffer_Create_New_TP_Connection_State."Create Connection" ("Action")) -> (s? t:f=w411:T22)
          }
          frame "Create Connection" {
            # "Stop if the intended address wasn't us."
            n131 = call-poly "Connnection Mode Buffer.vi"("CAN frame"=w432, "error in (no error)"=w434) -> ("Connection Cluster Out"=w431:T27, "error out"=w433:errorcluster)  [unwired: 12 out]
            n132 = call-poly "Connnection Mode Buffer.vi"("Connection Cluster"=w431, "Connections Ref"=w429, "State"=TP_Connections_List_State."Add", "error in (no error)"=w433) -> ("Connection Cluster Out"=w428:T27, "error out"=w435:errorcluster)  [unwired: 1 in, 9 out]
            n133 = Unbundle By Name(w428) -> ("Destination Address"=w424:u8)
            n134 = Search 1D Array(1D array=w425, element=w424) -> (index of element=w426:i32)  [unwired: 1 in]
            n135 = Greater Or Equal To 0?(x=w426) -> (x >= 0?=w423:bool)
            n136 = Not(x=w423) -> (.not. x?=w427:bool)
          }
          frame "Create CTS Frame" {
            # "Only send if the message was intended for our address."
            n137 = Unbundle By Name(w448) -> ("Source Address"=w454:u8, "Destination Address"=w453:u8, "PGN"=w452:u32, "Total Expected Packets"=w450:u8)
            n138 = call-poly "Connnection Mode Buffer.vi"("PGN"=w452, "Source Address"=w453, "Destination Address"=w454, "Number of Packets to Send"=w450, "Next Packet to Send"=u8 1, "error in (no error)"=w449) -> ("Arb ID"=w441:u32, "Data"=w440:u8[], "error out"=w444:errorcluster)  [unwired: 1 in, 6 out]
            n139 = Bundle(cluster=T20 {"Identifier"=0, "Data"=[]} ("Data to Send"), "Identifier"=w441, "Data"=w440) -> (w438:T20)
            n140 = Enqueue Element(queue=w442, element=w438, error in (no error)=w444) -> (error out=w443:errorcluster)  [unwired: 3 out]
          }
          frame "Abort New Connection" {
            n141 = call-poly "Connnection Mode Buffer.vi"("CAN frame"=w464, "error in (no error)"=w463) -> ("Connection Cluster Out"=w461:T27, "error out"=w462:errorcluster)  [unwired: 12 out]
            n142 = Unbundle By Name(w461) -> ("Source Address"=w460:u8, "Destination Address"=w456:u8, "PGN"=w459:u32)
            n143 = Search 1D Array(1D array=w457, element=w456) -> (index of element=w458:i32)  [unwired: 1 in]
            n144 = Greater Or Equal To 0?(x=w458) -> (x >= 0?=w455:bool)
            n145 = case shown="False" w455 {
              tunnel: w462 -> [w471 w482]
              tunnel: [w471 w478] -> w467
              tunnel: w466 -> [_ w475]
              tunnel: w460 -> [_ w474]
              tunnel: w456 -> [_ w473]
              tunnel: w459 -> [_ w472]
              frame False {
              }
              frame True {
                n146 = call-poly "Connnection Mode Buffer.vi"("Destination Address"=w474, "Source Address"=w473, "PGN"=w472, "error in (no error)"=w482) -> ("Arb ID"=w481:u32, "Data"=w480:u8[], "error out"=w479:errorcluster)  [unwired: 2 in, 7 out]
                n147 = Bundle(cluster=T20 {"Identifier"=0, "Data"=[]} ("Data to Send"), "Identifier"=w481, "Data"=w480) -> (w476:T20)
                n148 = Enqueue Element(queue=w475, element=w476, error in (no error)=w479) -> (error out=w478:errorcluster)  [unwired: 3 out]
              }
            }
          }
        }
      }
    }
    frame "TP.CM - CTS" {
      n149 = call-poly "Connection Mode Generation.vi"("CM Gen Ref"=w486, "State"=TP_Connections_List_State."Get", "error in (no error)"=w496) -> ("CM Gen Ref out"=w485:T5, "Connections"=w487:T28[], "error out"=w488:errorcluster)  [unwired: 2 in, 8 out]
      n150 = call-poly "Connection Mode Generation.vi"("Connections"=w487, "CAN frame"=w484, "error in (no error)"=w488) -> ("Connection Cluster"=w491:T28, "CAN frame out"=w494:T9, "Found?"=w493:bool, "Index"=w492:i32, "error out"=w490:errorcluster)  [unwired: 1 in, 7 out]
      n151 = case shown="False" w493 {
        tunnel: w490 -> [w505 w526]
        tunnel: w491 -> [_ w525]
        tunnel: [w500 w522] -> w495
        tunnel: w492 -> [_ w520]
        tunnel: w494 -> [w503 w519]
        tunnel: w485 -> [_ w518]
        tunnel: w483 -> [w504 _]
        frame False {
          n152 = call-poly "Connnection Mode Buffer.vi"("Connections Ref"=w504, "State"=TP_Connections_List_State."Get", "error in (no error)"=w505) -> ("Connections Ref out"=w497:T4, "Connections"=w507:T27[], "error out"=w508:errorcluster)  [unwired: 2 in, 8 out]
          n153 = call-poly "Connnection Mode Buffer.vi"("Connecctions"=w507, "CAN frame"=w503, "error in (no error)"=w508) -> ("Connection Cluster Out"=w498:T27, "Found?"=w502:bool, "Index"=w499:i32, "error out"=w501:errorcluster)  [unwired: 9 out]
          n154 = case shown="False" w502 {
            tunnel: w501 -> [w509 w517]
            tunnel: [w509 w516] -> w500
            tunnel: w499 -> [_ w515]
            tunnel: w498 -> [_ w512]
            tunnel: w497 -> [_ w514]
            frame False {
            }
            frame True {
              n155 = call "Tick Count"() -> ("Tick Count(mSec)"=w510:u32)
              n156 = Bundle By Name(cluster=w512, "Start Time"=w510) -> (w511:T27)
              n157 = call-poly "Connnection Mode Buffer.vi"("Connection Cluster"=w511, "Connections Ref"=w514, "State"=TP_Connections_List_State."Update", "index"=w515, "error in (no error)"=w517) -> ("error out"=w516:errorcluster)  [unwired: 10 out]
            }
          }
        }
        frame True {
          n158 = call-poly "Connection Mode Generation.vi"("Connection Cluster"=w525, "CAN frame"=w519, "error in (no error)"=w526) -> ("Connection Cluster Out"=w524:T28, "error out"=w523:errorcluster)  [unwired: 11 out]
          n159 = call-poly "Connection Mode Generation.vi"("Connection Cluster"=w524, "CM Gen Ref"=w518, "State"=TP_Connections_List_State."Update", "index"=w520, "error in (no error)"=w523) -> ("error out"=w522:errorcluster)  [unwired: 10 out]
        }
      }
    }
    frame "TP.CM - EndofMsgACK" {
      # "DLE NOTE - Technically, I should wait for this when acquiring a connection mode message from an address other than mine (I generate the message if my address is the one the message is intended for)."
      n160 = call-poly "Connection Mode Generation.vi"("CM Gen Ref"=w529, "State"=TP_Connections_List_State."Get", "error in (no error)"=w537) -> ("CM Gen Ref out"=w528:T5, "Connections"=w532:T28[], "error out"=w531:errorcluster)  [unwired: 2 in, 8 out]
      n161 = call-poly "Connection Mode Generation.vi"("Connections"=w532, "CAN frame"=w527, "error in (no error)"=w531) -> ("Found?"=w534:bool, "Index"=w535:i32, "error out"=w533:errorcluster)  [unwired: 1 in, 9 out]
      n162 = case shown="True" w534 {
        tunnel: w533 -> [w538 w543]
        tunnel: [w538 w542] -> w536
        tunnel: w535 -> [_ w540]
        tunnel: w528 -> [_ w539]
        frame False {
        }
        frame True {
          n163 = call-poly "Connection Mode Generation.vi"("CM Gen Ref"=w539, "State"=TP_Connections_List_State."Remove", "index"=w540, "error in (no error)"=w543) -> ("error out"=w542:errorcluster)  [unwired: 1 in, 10 out]
        }
      }
    }
    frame "TP.CM - Abort" {
      n164 = call-poly "Connnection Mode Buffer.vi"("Connections Ref"=w547, "State"=TP_Connections_List_State."Get", "error in (no error)"=w553) -> ("Connections Ref out"=w546:T4, "Connections"=w550:T27[], "error out"=w552:errorcluster)  [unwired: 2 in, 8 out]
      n165 = call-poly "Connnection Mode Buffer.vi"("Connecctions"=w550, "CAN frame"=w544, "error in (no error)"=w552) -> ("Found?"=w549:bool, "Index"=w548:i32, "error out"=w555:errorcluster)  [unwired: 1 in, 9 out]
      n166 = case shown="True" w549 {
        tunnel: w555 -> [w565 w577]
        tunnel: [w566 w576] -> w554
        tunnel: w548 -> [_ w574]
        tunnel: w544 -> [w564 _]
        tunnel: w546 -> [_ w573]
        tunnel: w545 -> [w557 _]
        frame False {
          n167 = call-poly "Connection Mode Generation.vi"("CM Gen Ref"=w557, "State"=TP_Connections_List_State."Get", "error in (no error)"=w565) -> ("CM Gen Ref out"=w556:T5, "Connections"=w560:T28[], "error out"=w559:errorcluster)  [unwired: 2 in, 8 out]
          n168 = call-poly "Connection Mode Generation.vi"("Connections"=w560, "CAN frame"=w564, "error in (no error)"=w559) -> ("Found?"=w562:bool, "Index"=w563:i32, "error out"=w561:errorcluster)  [unwired: 1 in, 9 out]
          n169 = case shown="True" w562 {
            tunnel: w561 -> [w567 w572]
            tunnel: [w567 w571] -> w566
            tunnel: w563 -> [_ w569]
            tunnel: w556 -> [_ w568]
            frame False {
            }
            frame True {
              n170 = call-poly "Connection Mode Generation.vi"("CM Gen Ref"=w568, "State"=TP_Connections_List_State."Remove", "index"=w569, "error in (no error)"=w572) -> ("error out"=w571:errorcluster)  [unwired: 1 in, 10 out]
            }
          }
        }
        frame True {
          n171 = call-poly "Connnection Mode Buffer.vi"("Connections Ref"=w573, "State"=TP_Connections_List_State."Remove", "index"=w574, "error in (no error)"=w577) -> ("error out"=w576:errorcluster)  [unwired: 1 in, 10 out]
        }
      }
    }
    frame "ACL" {
      # "DLE NOTE - This needs to be added to handle rejections."
      # "Address Claimed (ACL) Stub"
      n172 = Unbundle By Name(w580) -> ("identifier"=w581:u32, "payload"=w588:u8[])
      n173 = call-poly "Common Conversions.vi"("Arb ID"=w581) -> ("Source Address"=w578:u8)  [unwired: 11 in, 3 out]
      n174 = case shown="0..253" w578 {
        selector: w578 -> [_ w592]
        tunnel: w589 -> [w590 w597]
        tunnel: [w590 w591] -> w583
        tunnel: w588 -> [_ w595]
        tunnel: w587 -> [_ w593]
        frame Default {
        }
        frame 0..253 {
          n175 = Bundle By Name(cluster=T23 {"Name"=[], "Address"=0} ("Data"), "Address"=w592, "Name"=w595) -> (w594:T23)
          n176 = call "Network Address Lookup Table.vi"("Action"=Address_Lookup_Table_Action."Add", "error in (no error)"=w597, "Address"=w592, "Data"=w594, "Address LUT"=w593) -> ("error out"=w591:errorcluster)  [unwired: 2 in, 4 out]
        }
      }
      n177 = And(x=w581, y=u32 536870911) -> (x .and. y?=w584:u32)
      n178 = Bundle By Name(cluster=w580, "identifier"=w584) -> (w585:T9)
      n179 = Enqueue Element(queue=w579, element=w585, error in (no error)=w583) -> (error out=w582:errorcluster)  [unwired: 3 out]
    }
    frame "PDU 2", "Proprietary B" {
      # "Global PDUs (PDU2)"
      n180 = Unbundle By Name(w599) -> ("identifier"=w606:u32)
      n181 = And(x=w606, y=u32 536870911) -> (x .and. y?=w603:u32)
      n182 = Bundle By Name(cluster=w599, "identifier"=w603) -> (w604:T9)
      n183 = Enqueue Element(queue=w600, element=w604, error in (no error)=w601) -> (error out=w602:errorcluster)  [unwired: 3 out]
    }
    frame "TP.CM - Error", "Error" {
      # "Proprietary B Stub"
    }
  }
  "error out" <- w19
